vi "Initialize.vi"(8 "error in":errorcluster, 9 "Number of Channels":u32=1, 10 "Plugin Name":string, 11 "Cycler in":refnum<class "Cycler.lvclass">) -> (0 "error out":errorcluster, 3 "Cycler out":refnum<class "Cycler.lvclass">)   [LabVIEW 2023, in "Cycler.lvclass"]
doc: "This VI initializes required data channels for a Cycler. Wire the number of power output channels to <b>Number of Channels</b>, the default is 1."
uses:
  Cycler.lvclass
  Cycler.lvclass/Cycler.ctl
  <vilib>/ADAS Replay HIL/Channels/Tag Wrapper/Polymorphic/Open Producer Tag (Double).vi
  <vilib>/ADAS Replay HIL/Channels/Tag Wrapper/Polymorphic/Set Default Value (Double).vi
  <vilib>/ADAS Replay HIL/Channels/Tag Wrapper/Polymorphic/Open Consumer Tag (Boolean).vi
  <vilib>/ADAS Replay HIL/Channels/Tag Wrapper/Polymorphic/Set Default Value (Boolean).vi
  <vilib>/ADAS Replay HIL/Channels/Tag Wrapper/Polymorphic/Open Producer Tag (I32).vi
  <vilib>/ADAS Replay HIL/Channels/Tag Wrapper/Polymorphic/Set Default Value (I32).vi
  <vilib>/ADAS Replay HIL/Channels/Tag Wrapper/Polymorphic/Open Producer Tag (Boolean).vi
  <vilib>/ADAS Replay HIL/Channels/Tag Wrapper/Polymorphic/Open Producer Tag (Double).vi/45cd6eaa-a1ce-41a4-8aba-62a49d103d7e.vi
  <vilib>/ADAS Replay HIL/Channels/Tag Wrapper/Polymorphic/Set Default Value (Double).vi/228e99de-6fcf-414d-86fc-dc277c7b351f.vi
  <vilib>/ADAS Replay HIL/Channels/Tag Wrapper/Polymorphic/Open Consumer Tag (Boolean).vi/bacb721e-673a-491a-accd-959f2e1f334e.vi
  <vilib>/ADAS Replay HIL/Channels/Tag Wrapper/Polymorphic/Set Default Value (Boolean).vi/228e99de-6fcf-414d-86fc-dc277c7b351f.vi
  <vilib>/ADAS Replay HIL/Channels/Tag Wrapper/Polymorphic/Open Producer Tag (I32).vi/45cd6eaa-a1ce-41a4-8aba-62a49d103d7e.vi
  <vilib>/ADAS Replay HIL/Channels/Tag Wrapper/Polymorphic/Set Default Value (I32).vi/228e99de-6fcf-414d-86fc-dc277c7b351f.vi
  <vilib>/ADAS Replay HIL/Channels/Tag Wrapper/Polymorphic/Open Producer Tag (Boolean).vi/45cd6eaa-a1ce-41a4-8aba-62a49d103d7e.vi
  <vilib>/ADAS Replay HIL/Channels/Tag Wrapper/Polymorphic/Open Producer Tag (Double).vi/45cd6eaa-a1ce-41a4-8aba-62a49d103d7e.vi/c28b0ead-42ad-4072-80a2-aca7f2bd7ce3.vi
  <vilib>/ADAS Replay HIL/Channels/Tag Wrapper/Polymorphic/Set Default Value (Double).vi/228e99de-6fcf-414d-86fc-dc277c7b351f.vi/4bc1c15b-36ab-481f-b8dd-c64075ce723a.vi
  <vilib>/ADAS Replay HIL/Channels/Tag Wrapper/Polymorphic/Open Consumer Tag (Boolean).vi/bacb721e-673a-491a-accd-959f2e1f334e.vi/c28b0ead-42ad-4072-80a2-aca7f2bd7ce3.vi
  <vilib>/ADAS Replay HIL/Channels/Tag Wrapper/Polymorphic/Set Default Value (Boolean).vi/228e99de-6fcf-414d-86fc-dc277c7b351f.vi/4bc1c15b-36ab-481f-b8dd-c64075ce723a.vi
  <vilib>/ADAS Replay HIL/Channels/Tag Wrapper/Polymorphic/Open Producer Tag (I32).vi/45cd6eaa-a1ce-41a4-8aba-62a49d103d7e.vi/c28b0ead-42ad-4072-80a2-aca7f2bd7ce3.vi
  <vilib>/ADAS Replay HIL/Channels/Tag Wrapper/Polymorphic/Set Default Value (I32).vi/228e99de-6fcf-414d-86fc-dc277c7b351f.vi/4bc1c15b-36ab-481f-b8dd-c64075ce723a.vi
  <vilib>/ADAS Replay HIL/Channels/Tag Wrapper/Polymorphic/Open Producer Tag (Boolean).vi/45cd6eaa-a1ce-41a4-8aba-62a49d103d7e.vi/c28b0ead-42ad-4072-80a2-aca7f2bd7ce3.vi
  <vilib>/ADAS Replay HIL/AdasHilServices/AdasHilServices Fill In Error Info Ex.vi
  <vilib>/ADAS Replay HIL/Channels/Tag Wrapper/Tag Wrapper.lvlib
  Utilities/Utilities.lvlib
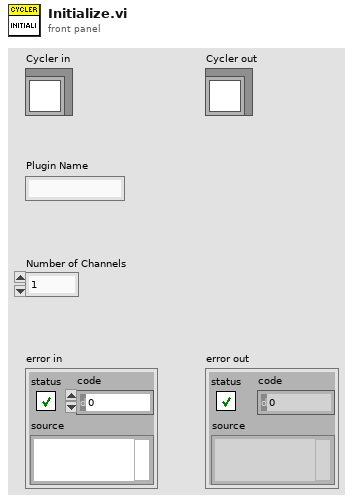
[diagram p1: front panel]
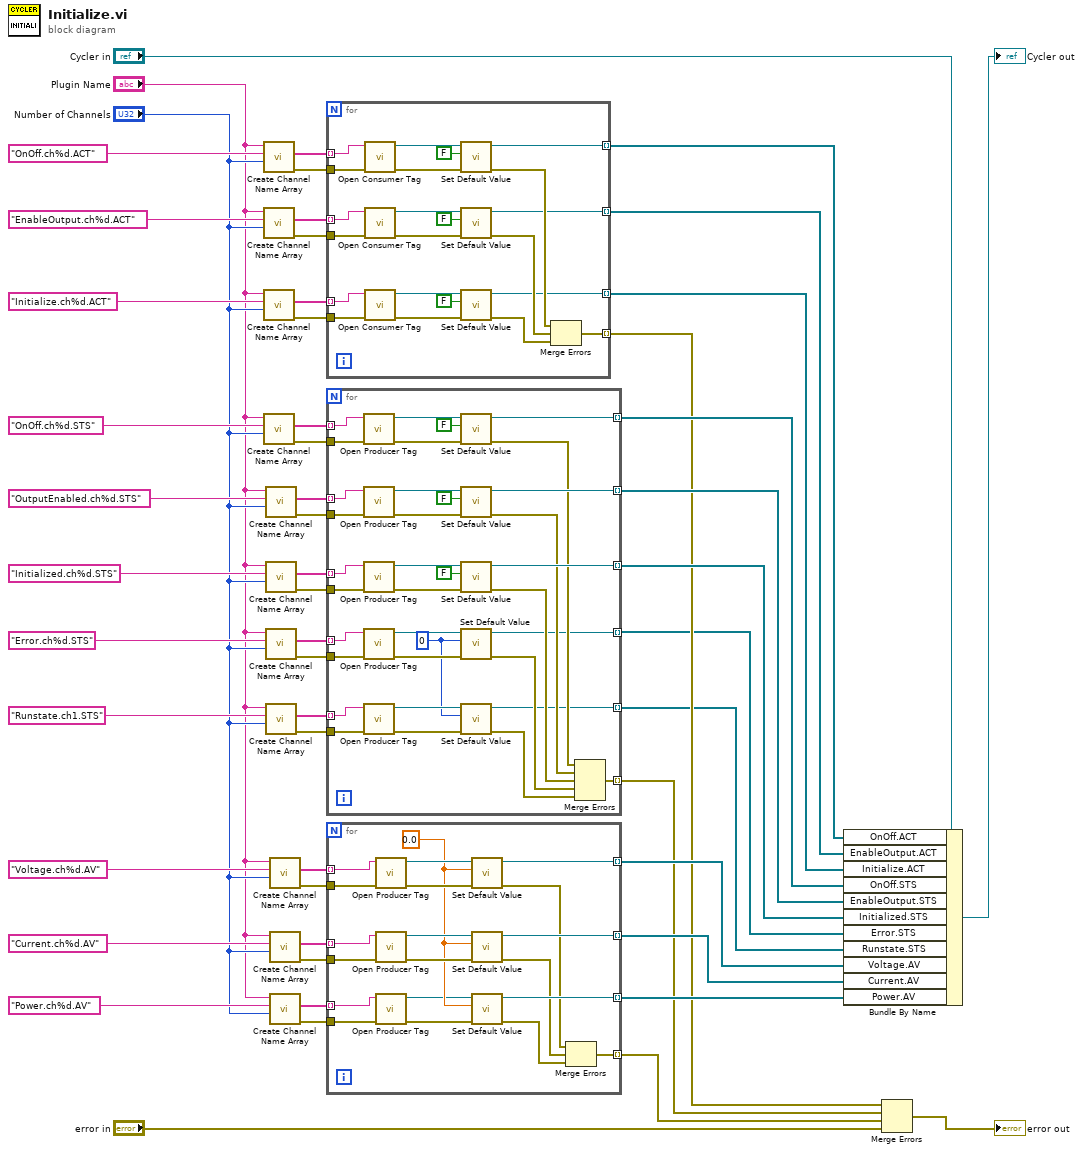
[diagram p0: block diagram]
diagram:
  n1 = call "Create Channel Name Array.vi"("Number of Channels"="Number of Channels", "Channel Format String"="OnOff.ch%d.ACT", "Plugin Name"="Plugin Name") -> ("error out"=w49:errorcluster, "Channel Names"=w52:string[])  [unwired: 7 in]
  n2 = call "Create Channel Name Array.vi"("Number of Channels"="Number of Channels", "Channel Format String"="EnableOutput.ch%d.ACT", "Plugin Name"="Plugin Name") -> ("error out"=w47:errorcluster, "Channel Names"=w46:string[])  [unwired: 7 in]
  n3 = call "Create Channel Name Array.vi"("Number of Channels"="Number of Channels", "Channel Format String"="Initialize.ch%d.ACT", "Plugin Name"="Plugin Name") -> ("error out"=w12:errorcluster, "Channel Names"=w13:string[])  [unwired: 7 in]
  n4 = call "Create Channel Name Array.vi"("Number of Channels"="Number of Channels", "Channel Format String"="OnOff.ch%d.STS", "Plugin Name"="Plugin Name") -> ("error out"=w44:errorcluster, "Channel Names"=w45:string[])  [unwired: 7 in]
  n5 = call "Create Channel Name Array.vi"("Number of Channels"="Number of Channels", "Channel Format String"="OutputEnabled.ch%d.STS", "Plugin Name"="Plugin Name") -> ("error out"=w48:errorcluster, "Channel Names"=w51:string[])  [unwired: 7 in]
  n6 = call "Create Channel Name Array.vi"("Number of Channels"="Number of Channels", "Channel Format String"="Initialized.ch%d.STS", "Plugin Name"="Plugin Name") -> ("error out"=w39:errorcluster, "Channel Names"=w37:string[])  [unwired: 7 in]
  n7 = call "Create Channel Name Array.vi"("Number of Channels"="Number of Channels", "Channel Format String"="Error.ch%d.STS", "Plugin Name"="Plugin Name") -> ("error out"=w7:errorcluster, "Channel Names"=w5:string[])  [unwired: 7 in]
  n8 = call "Create Channel Name Array.vi"("Number of Channels"="Number of Channels", "Channel Format String"="Runstate.ch1.STS", "Plugin Name"="Plugin Name") -> ("error out"=w8:errorcluster, "Channel Names"=w10:string[])  [unwired: 7 in]
  n9 = call "Create Channel Name Array.vi"("Number of Channels"="Number of Channels", "Channel Format String"="Voltage.ch%d.AV", "Plugin Name"="Plugin Name") -> ("error out"=w30:errorcluster, "Channel Names"=w31:string[])  [unwired: 7 in]
  n10 = call "Create Channel Name Array.vi"("Number of Channels"="Number of Channels", "Channel Format String"="Current.ch%d.AV", "Plugin Name"="Plugin Name") -> ("error out"=w28:errorcluster, "Channel Names"=w29:string[])  [unwired: 7 in]
  n11 = call "Create Channel Name Array.vi"("Number of Channels"="Number of Channels", "Channel Format String"="Power.ch%d.AV", "Plugin Name"="Plugin Name") -> ("error out"=w26:errorcluster, "Channel Names"=w27:string[])  [unwired: 7 in]
  n12 = for {
    tunnel: w52 -> [w75] mode=indexing
    tunnel: w49 -> [w74]
    tunnel: w47 -> [w73]
    tunnel: w46 -> [w72] mode=indexing
    tunnel: [w63] -> w19 mode=indexing
    tunnel: [w62] -> w18 mode=indexing
    tunnel: [w61] -> w17 mode=indexing
    tunnel: w12 -> [w56]
    tunnel: w13 -> [w57] mode=indexing
    tunnel: [w54] -> w11 mode=indexing
    n13 = call-poly <vilib>:"Open Consumer Tag.vi"("error in"=w74, "Channel Name"=w75) -> ("error out"=w70:errorcluster, "ADAS HIL Channel"=w71:refnum<k21>)  [unwired: 8 in]
    n14 = call-poly <vilib>:"Open Consumer Tag.vi"("error in"=w73, "Channel Name"=w72) -> ("error out"=w68:errorcluster, "ADAS HIL Channel"=w69:refnum<k21>)  [unwired: 8 in]
    n15 = call-poly <vilib>:"Open Consumer Tag.vi"("error in"=w56, "Channel Name"=w57) -> ("error out"=w59:errorcluster, "ADAS HIL Channel"=w58:refnum<k21>)  [unwired: 8 in]
    n16 = call-poly <vilib>:"Set Default Value.vi"("error in"=w70, "Default Value"=FALSE, "ADAS HIL Channel in"=w71) -> ("error out"=w65:errorcluster, "ADAS HIL Channel out"=w62:refnum<k21>)  [unwired: 7 in]
    n17 = call-poly <vilib>:"Set Default Value.vi"("error in"=w68, "Default Value"=FALSE, "ADAS HIL Channel in"=w69) -> ("error out"=w64:errorcluster, "ADAS HIL Channel out"=w63:refnum<k21>)  [unwired: 7 in]
    n18 = call-poly <vilib>:"Set Default Value.vi"("error in"=w59, "Default Value"=FALSE, "ADAS HIL Channel in"=w58) -> ("error out"=w55:errorcluster, "ADAS HIL Channel out"=w54:refnum<k21>)  [unwired: 7 in]
    n19 = Merge Errors(w65, w64, w55) -> (w61:errorcluster)
  }
  n20 = for {
    tunnel: w51 -> [w110] mode=indexing
    tunnel: w48 -> [w109]
    tunnel: w45 -> [w108] mode=indexing
    tunnel: w44 -> [w107]
    tunnel: w39 -> [w106]
    tunnel: w37 -> [w105] mode=indexing
    tunnel: [w95] -> w20 mode=indexing
    tunnel: [w94] -> w21 mode=indexing
    tunnel: [w93] -> w22 mode=indexing
    tunnel: [w89] -> w16 mode=indexing
    tunnel: w5 -> [w81] mode=indexing
    tunnel: w7 -> [w82]
    tunnel: w8 -> [w83]
    tunnel: w10 -> [w84] mode=indexing
    tunnel: [w77] -> w2 mode=indexing
    tunnel: [w76] -> w1 mode=indexing
    w80 = 0 ("Default Value")
    n21 = call-poly <vilib>:"Open Producer Tag.vi"("error in"=w107, "Channel Name"=w108) -> ("error out"=w99:errorcluster, "ADAS HIL Channel"=w100:refnum<k21>)  [unwired: 8 in]
    n22 = call-poly <vilib>:"Open Producer Tag.vi"("error in"=w109, "Channel Name"=w110) -> ("error out"=w102:errorcluster, "ADAS HIL Channel"=w101:refnum<k21>)  [unwired: 8 in]
    n23 = call-poly <vilib>:"Open Producer Tag.vi"("error in"=w106, "Channel Name"=w105) -> ("error out"=w104:errorcluster, "ADAS HIL Channel"=w103:refnum<k21>)  [unwired: 8 in]
    n24 = call-poly <vilib>:"Open Producer Tag.vi"("error in"=w82, "Channel Name"=w81) -> ("error out"=w87:errorcluster, "ADAS HIL Channel"=w88:refnum<k21>)  [unwired: 8 in]
    n25 = call-poly <vilib>:"Open Producer Tag.vi"("error in"=w83, "Channel Name"=w84) -> ("error out"=w85:errorcluster, "ADAS HIL Channel"=w86:refnum<k21>)  [unwired: 8 in]
    n26 = call-poly <vilib>:"Set Default Value.vi"("error in"=w99, "Default Value"=FALSE, "ADAS HIL Channel in"=w100) -> ("error out"=w92:errorcluster, "ADAS HIL Channel out"=w95:refnum<k21>)  [unwired: 7 in]
    n27 = call-poly <vilib>:"Set Default Value.vi"("error in"=w102, "Default Value"=FALSE, "ADAS HIL Channel in"=w101) -> ("error out"=w91:errorcluster, "ADAS HIL Channel out"=w94:refnum<k21>)  [unwired: 7 in]
    n28 = call-poly <vilib>:"Set Default Value.vi"("error in"=w104, "Default Value"=FALSE, "ADAS HIL Channel in"=w103) -> ("error out"=w90:errorcluster, "ADAS HIL Channel out"=w93:refnum<k21>)  [unwired: 7 in]
    n29 = call-poly <vilib>:"Set Default Value.vi"("error in"=w87, "Default Value"=w80, "ADAS HIL Channel in"=w88) -> ("error out"=w79:errorcluster, "ADAS HIL Channel out"=w76:refnum<k21>)  [unwired: 7 in]
    n30 = call-poly <vilib>:"Set Default Value.vi"("error in"=w85, "Default Value"=w80, "ADAS HIL Channel in"=w86) -> ("error out"=w78:errorcluster, "ADAS HIL Channel out"=w77:refnum<k21>)  [unwired: 7 in]
    n31 = Merge Errors(w92, w91, w90, w79, w78) -> (w89:errorcluster)
  }
  n32 = for {
    tunnel: w31 -> [w130] mode=indexing
    tunnel: [w128] -> w25 mode=indexing
    tunnel: w30 -> [w127]
    tunnel: w29 -> [w125] mode=indexing
    tunnel: w28 -> [w124]
    tunnel: [w122] -> w24 mode=indexing
    tunnel: w27 -> [w118] mode=indexing
    tunnel: w26 -> [w117]
    tunnel: [w115] -> w23 mode=indexing
    tunnel: [w111] -> w15 mode=indexing
    w120 = 0.0 ("Default Value")
    n33 = call-poly <vilib>:"Open Producer Tag.vi"("error in"=w127, "Channel Name"=w130) -> ("error out"=w126:errorcluster, "ADAS HIL Channel"=w129:refnum<k21>)  [unwired: 8 in]
    n34 = call-poly <vilib>:"Open Producer Tag.vi"("error in"=w124, "Channel Name"=w125) -> ("error out"=w121:errorcluster, "ADAS HIL Channel"=w123:refnum<k21>)  [unwired: 8 in]
    n35 = call-poly <vilib>:"Open Producer Tag.vi"("error in"=w117, "Channel Name"=w118) -> ("error out"=w116:errorcluster, "ADAS HIL Channel"=w119:refnum<k21>)  [unwired: 8 in]
    n36 = call-poly <vilib>:"Set Default Value.vi"("error in"=w126, "Default Value"=w120, "ADAS HIL Channel in"=w129) -> ("error out"=w114:errorcluster, "ADAS HIL Channel out"=w128:refnum<k21>)  [unwired: 7 in]
    n37 = call-poly <vilib>:"Set Default Value.vi"("error in"=w121, "Default Value"=w120, "ADAS HIL Channel in"=w123) -> ("error out"=w113:errorcluster, "ADAS HIL Channel out"=w122:refnum<k21>)  [unwired: 7 in]
    n38 = call-poly <vilib>:"Set Default Value.vi"("error in"=w116, "Default Value"=w120, "ADAS HIL Channel in"=w119) -> ("error out"=w112:errorcluster, "ADAS HIL Channel out"=w115:refnum<k21>)  [unwired: 7 in]
    n39 = Merge Errors(w114, w113, w112) -> (w111:errorcluster)
  }
  n40 = Bundle By Name(cluster="Cycler in", "OnOff.ACT"=w18, "EnableOutput.ACT"=w19, "Initialize.ACT"=w11, "OnOff.STS"=w20, "EnableOutput.STS"=w21, "Initialized.STS"=w22, "Error.STS"=w1, "Runstate.STS"=w2, "Voltage.AV"=w25, "Current.AV"=w24, "Power.AV"=w23) -> (→"Cycler out":refnum<class "Cycler.lvclass">)
  n41 = Merge Errors(w17, w16, w15, "error in") -> (→"error out":errorcluster)
